vi "Update Categories.vi"(8 "error in (no error)":errorcluster, 11 "VIStore in":refnum<class "VIStore.lvclass">) -> (0 "error out":errorcluster, 3 "VIStore out":refnum<class "VIStore.lvclass">)   [LabVIEW 2015, in "VI App Store.lvlib" / "VIStore.lvclass"]
uses:
  VIStore.lvclass
  VIStore.lvclass/VIStore.ctl
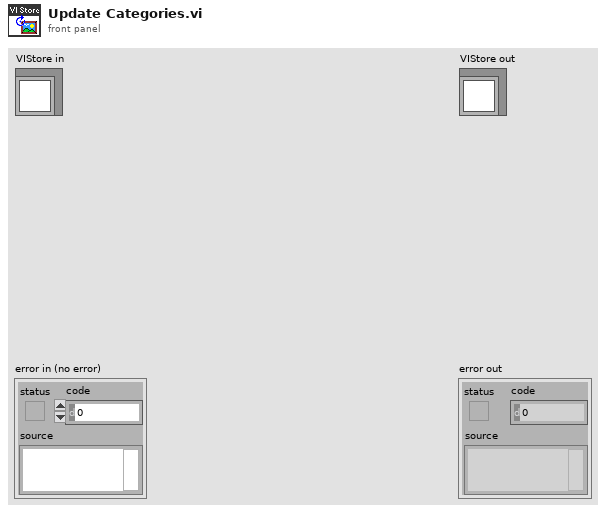
[diagram p1: front panel]
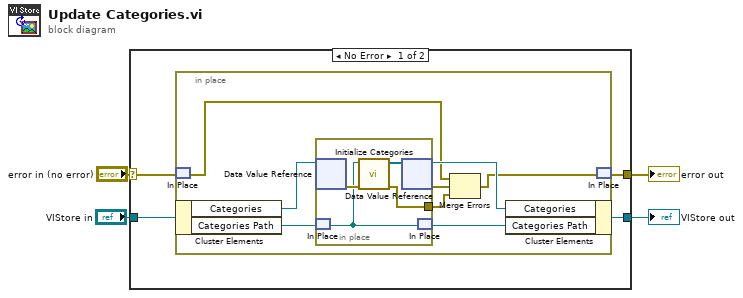
[diagram p0: block diagram]
diagram:
  n1 = case shown="No Error" "error in (no error)" {
    selector: "error in (no error)" -> [w6 w22]
    tunnel: [w5 w22] -> w3
    tunnel: [w8 w21] -> w1
    tunnel: "VIStore in" -> [w7 w21]
    frame No Error {
      n2 = in-place {
        n3 = in-place-match #1(w6) -> (w9:errorcluster)
        n4 = in-place-cluster #2(w7) -> ("Categories"=w16:refnum<data-value>, "Categories Path"=w10:path)
        n5 = in-place {
          in-place-border: [w18] -> w13
          n6 = in-place-dvr #3(w16) -> (w19:errorcluster)  [unwired: 1 out]
          n7 = in-place-match #4(w10) -> (w17:path)
          n8 = call "Initialize Categories.vi"("error in (no error)"=w19, "Cats XML"=w17) -> ("error out"=w18:errorcluster, "All Categories"=w20:refnum<class "Category.lvclass">[])  [unwired: 8 in]
          n9 = in-place-dvr #3(w20) -> (w15:refnum<data-value>, w14:errorcluster)
          n10 = in-place-match #4(w17) -> (w12:path)
        }
        n11 = Merge Errors(w9, w14, w13) -> (w11:errorcluster)
        n12 = in-place-cluster #2("Categories"=w15, "Categories Path"=w12) -> (w8:refnum<class "VIStore.lvclass">)
        n13 = in-place-match #1(w11) -> (w5:errorcluster)
      }
    }
    frame Error {
    }
  }
  "error out" <- w3
  "VIStore out" <- w1
